vi "LakeShore218_Status.vi"() -> (1 "n_ng":u8, 2 "value2":T1, 3 "value1":T2)   [LabVIEW 2019]
uses:
  LakeShore218_Global.vi
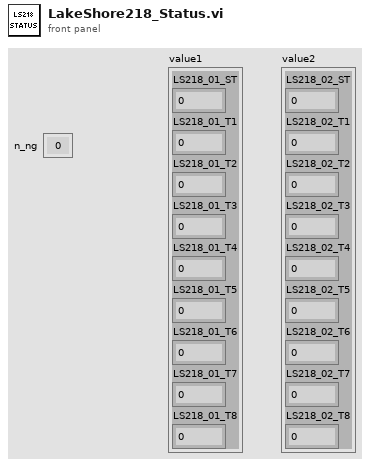
[diagram p1: front panel]
types:
  T1 = cluster{"LS218_02_ST":u32, "LS218_02_T1":dbl, "LS218_02_T2":dbl, "LS218_02_T3":dbl, "LS218_02_T4":dbl, "LS218_02_T5":dbl, "LS218_02_T6":dbl, "LS218_02_T7":dbl, "LS218_02_T8":dbl}
  T2 = cluster{"LS218_01_ST":u32, "LS218_01_T1":dbl, "LS218_01_T2":dbl, "LS218_01_T3":dbl, "LS218_01_T4":dbl, "LS218_01_T5":dbl, "LS218_01_T6":dbl, "LS218_01_T7":dbl, "LS218_01_T8":dbl}
  T3 = enum32{"Bad", "Idle", "Run top level", "Running"}
  T4 = cluster{"MKS670_1000_ST":u32, "LS218_02_T1":dbl, "LS218_02_T2":dbl, "LS218_02_T3":dbl, "LS218_02_T4":dbl, "LS218_02_T5":dbl, "LS218_02_T6":dbl, "LS218_02_T7":dbl, "LS218_02_T8":dbl}
  T5 = cluster{"MKS670_1000_ST":u32, "LS218_01_T1":dbl, "LS218_01_T2":dbl, "LS218_01_T3":dbl, "LS218_01_T4":dbl, "LS218_01_T5":dbl, "LS218_01_T6":dbl, "LS218_01_T7":dbl, "LS218_01_T8":dbl}
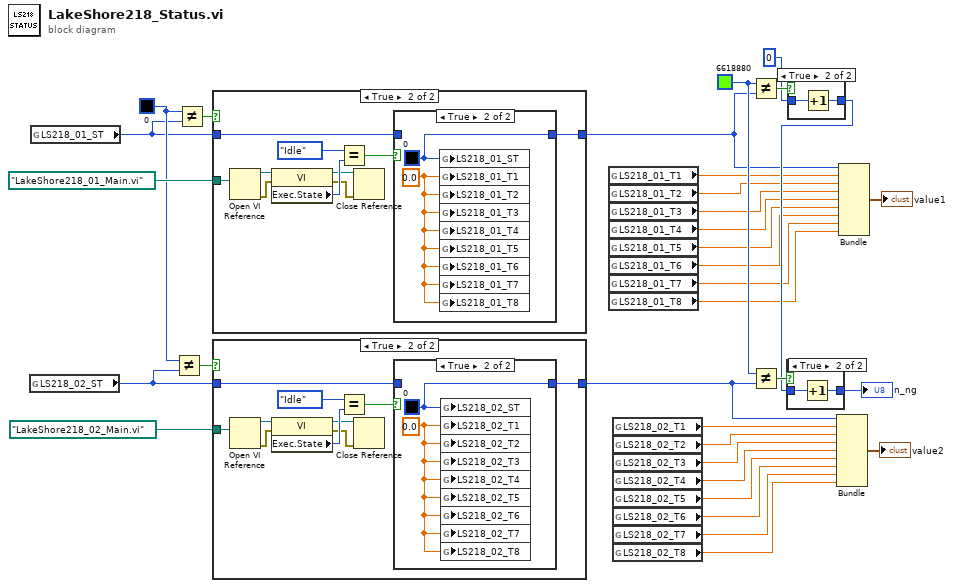
[diagram p0: block diagram]
diagram:
  w28 = u32 6618880 ("MKS670_1000_ST 2")
  w29 = u32 0 ("MKS670_1000_ST 2")
  n1 = global read "LakeShore218_Global.vi" "LS218_02_ST"() -> (w22:u32)
  n2 = global read "LakeShore218_Global.vi" "LS218_01_ST"() -> (w23:u32)
  n3 = Not Equal?(x=w29, y=w22) -> (x != y?=w31:bool)
  n4 = Not Equal?(x=w29, y=w23) -> (x != y?=w33:bool)
  n5 = case shown="True" w33 {
    tunnel: w23 -> [w34 w36]
    tunnel: [w34 w35] -> w20
    tunnel: path "LakeShore218_01_Main.vi" ("vi path") -> [_ w37]
    frame False {
    }
    frame True {
      n6 = Open VI Reference(vi path=w37) -> (vi reference=w44:refnum<vi>, error out=w43:errorcluster)  [unwired: 5 in]
      n7 = property class="VI"(reference=w44, error in=w43) -> (reference out=w39:refnum<vi>, error out=w38:errorcluster, "Exec.State"=w41:T3)
      n8 = Equal?(x=T3."Idle" ("Execution:State"), y=w41) -> (x = y?=w42:bool)
      n9 = Close Reference(reference=w39, error in (no error)=w38) -> ()  [unwired: 1 out]
      n10 = case shown="True" w42 {
        tunnel: w36 -> [w45 _]
        tunnel: [w45 w47] -> w35
        frame False {
        }
        frame True {
          w46 = 0.0 ("MKS670_1000_P")
          w47 = u32 0 ("MKS670_1000_ST")
          n11 = global write "LakeShore218_Global.vi" "LS218_01_ST"(w47) -> ()
          n12 = global write "LakeShore218_Global.vi" "LS218_01_T1"(w46) -> ()
          n13 = global write "LakeShore218_Global.vi" "LS218_01_T2"(w46) -> ()
          n14 = global write "LakeShore218_Global.vi" "LS218_01_T3"(w46) -> ()
          n15 = global write "LakeShore218_Global.vi" "LS218_01_T4"(w46) -> ()
          n16 = global write "LakeShore218_Global.vi" "LS218_01_T5"(w46) -> ()
          n17 = global write "LakeShore218_Global.vi" "LS218_01_T6"(w46) -> ()
          n18 = global write "LakeShore218_Global.vi" "LS218_01_T7"(w46) -> ()
          n19 = global write "LakeShore218_Global.vi" "LS218_01_T8"(w46) -> ()
        }
      }
    }
  }
  n20 = case shown="True" w31 {
    tunnel: w22 -> [w48 w50]
    tunnel: [w48 w49] -> w11
    tunnel: path "LakeShore218_02_Main.vi" ("vi path") -> [_ w51]
    frame False {
    }
    frame True {
      n21 = Open VI Reference(vi path=w51) -> (vi reference=w58:refnum<vi>, error out=w57:errorcluster)  [unwired: 5 in]
      n22 = property class="VI"(reference=w58, error in=w57) -> (reference out=w53:refnum<vi>, error out=w52:errorcluster, "Exec.State"=w55:T3)
      n23 = Equal?(x=T3."Idle" ("Execution:State"), y=w55) -> (x = y?=w56:bool)
      n24 = Close Reference(reference=w53, error in (no error)=w52) -> ()  [unwired: 1 out]
      n25 = case shown="True" w56 {
        tunnel: w50 -> [w59 _]
        tunnel: [w59 w61] -> w49
        frame False {
        }
        frame True {
          w60 = 0.0 ("MKS670_1000_P")
          w61 = u32 0 ("MKS670_1000_ST")
          n26 = global write "LakeShore218_Global.vi" "LS218_02_ST"(w61) -> ()
          n27 = global write "LakeShore218_Global.vi" "LS218_02_T1"(w60) -> ()
          n28 = global write "LakeShore218_Global.vi" "LS218_02_T2"(w60) -> ()
          n29 = global write "LakeShore218_Global.vi" "LS218_02_T3"(w60) -> ()
          n30 = global write "LakeShore218_Global.vi" "LS218_02_T4"(w60) -> ()
          n31 = global write "LakeShore218_Global.vi" "LS218_02_T5"(w60) -> ()
          n32 = global write "LakeShore218_Global.vi" "LS218_02_T6"(w60) -> ()
          n33 = global write "LakeShore218_Global.vi" "LS218_02_T7"(w60) -> ()
          n34 = global write "LakeShore218_Global.vi" "LS218_02_T8"(w60) -> ()
        }
      }
    }
  }
  n35 = global read "LakeShore218_Global.vi" "LS218_01_T1"() -> (w19:dbl)
  n36 = global read "LakeShore218_Global.vi" "LS218_01_T2"() -> (w17:dbl)
  n37 = global read "LakeShore218_Global.vi" "LS218_01_T3"() -> (w18:dbl)
  n38 = global read "LakeShore218_Global.vi" "LS218_01_T4"() -> (w16:dbl)
  n39 = global read "LakeShore218_Global.vi" "LS218_01_T5"() -> (w15:dbl)
  n40 = global read "LakeShore218_Global.vi" "LS218_01_T6"() -> (w14:dbl)
  n41 = global read "LakeShore218_Global.vi" "LS218_01_T7"() -> (w13:dbl)
  n42 = global read "LakeShore218_Global.vi" "LS218_01_T8"() -> (w12:dbl)
  n43 = global read "LakeShore218_Global.vi" "LS218_02_T1"() -> (w10:dbl)
  n44 = global read "LakeShore218_Global.vi" "LS218_02_T2"() -> (w9:dbl)
  n45 = global read "LakeShore218_Global.vi" "LS218_02_T3"() -> (w8:dbl)
  n46 = global read "LakeShore218_Global.vi" "LS218_02_T4"() -> (w7:dbl)
  n47 = global read "LakeShore218_Global.vi" "LS218_02_T5"() -> (w6:dbl)
  n48 = global read "LakeShore218_Global.vi" "LS218_02_T6"() -> (w5:dbl)
  n49 = global read "LakeShore218_Global.vi" "LS218_02_T7"() -> (w4:dbl)
  n50 = global read "LakeShore218_Global.vi" "LS218_02_T8"() -> (w3:dbl)
  n51 = Not Equal?(x=w28, y=w20) -> (x != y?=w27:bool)
  n52 = Not Equal?(x=w28, y=w11) -> (x != y?=w25:bool)
  n53 = case shown="True" w27 {
    tunnel: u8 0 ("n_idle") -> [w62 w64]
    tunnel: [w62 w63] -> w24
    frame False {
    }
    frame True {
      n54 = Increment(x=w64) -> (x+1=w63:u8)
    }
  }
  n55 = case shown="True" w25 {
    tunnel: w24 -> [w65 w67]
    tunnel: [w65 w66] -> w21
    frame False {
    }
    frame True {
      n56 = Increment(x=w67) -> (x+1=w66:u8)
    }
  }
  "n_ng" <- w21
  n57 = Bundle("MKS670_1000_ST"=w11, "LS218_02_T1"=w10, "LS218_02_T2"=w9, "LS218_02_T3"=w8, "LS218_02_T4"=w7, "LS218_02_T5"=w6, "LS218_02_T6"=w5, "LS218_02_T7"=w4, "LS218_02_T8"=w3) -> (→"value2":T4)  [unwired: 1 in]
  n58 = Bundle("MKS670_1000_ST"=w20, "LS218_01_T1"=w19, "LS218_01_T2"=w17, "LS218_01_T3"=w18, "LS218_01_T4"=w16, "LS218_01_T5"=w15, "LS218_01_T6"=w14, "LS218_01_T7"=w13, "LS218_01_T8"=w12) -> (→"value1":T5)  [unwired: 1 in]
